vi "WriteIQ_int16.vi"(8 "error in (no error)":errorcluster, 9 "dt":dbl=1.0, 10 "data":i16[](array[numeric]), 11 "reference in":refnum<class "mmWave data.lvclass">) -> (0 "error out":errorcluster, 3 "reference out":refnum<class "mmWave data.lvclass">)   [LabVIEW 2019, in "mmWave data.lvclass"]
doc: "Writes IQ data as I16 waveform"
uses:
  mmWave data.lvclass
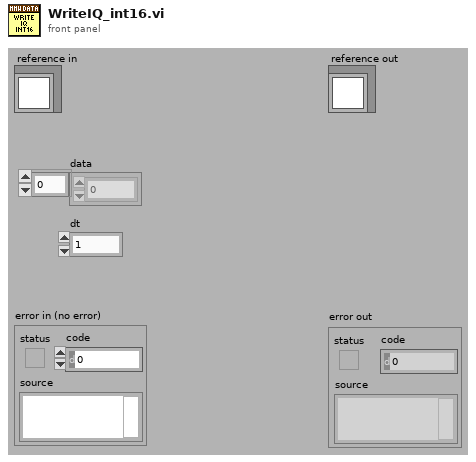
[diagram p1: front panel]
types:
  T1 = typedef "mmWave data.lvclass/ObjectAttributes.ctl" = cluster{"MyAttribute":dbl, "size":i32}
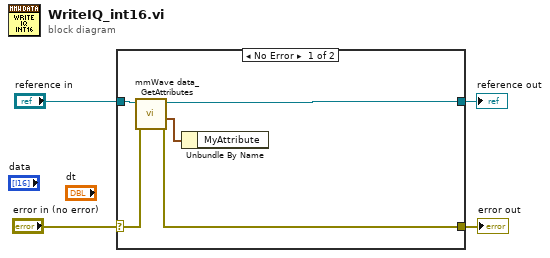
[diagram p0: block diagram]
diagram:
  n1 = case shown="No Error" "error in (no error)" {
    selector: "error in (no error)" -> [w9 w11]
    tunnel: [w8 w11] -> w3
    tunnel: [w7 w10] -> w1
    tunnel: "reference in" -> [w5 w10]
    frame No Error {
      n2 = call "mmWave data_GetAttributes.vi"("error in (no error)"=w9, "reference in"=w5) -> ("error out"=w8:errorcluster, "attributes"=w6:T1, "reference out"=w7:refnum<class "mmWave data.lvclass">)  [unwired: 6 in, 1 out]
      n3 = Unbundle By Name(w6) -> ()  [unwired: 1 out]
    }
    frame Error {
    }
  }
  "error out" <- w3
  "reference out" <- w1
